vi "DSP 1st.vi"(0 "Input Signal":dbl[](array[numeric]), 1 "Work position parameter":i32[](array[numeric]), 2 "Minus Noise(F : Don't)":bool, 3 "Smooth(F : Don't)":bool, 5 "RF Window":dbl[](array[numeric]), 7 "IIR Filter Cluster":T1 caption="IIR滤波器簇" {"Forward Coefficients" format="%.4f"; "Reverse Coefficients" format="%.4f"}, 9 "Noise Signal":dbl[](array[numeric]), 11 "error in (no error)":errorcluster caption="错误输入（无错误）", 12 "SPAN":i32, 13 "Logarithmic Base":dbl) -> (4 "DSP signal":dbl[](array[numeric]), 15 "error out":errorcluster caption="错误输出")   [LabVIEW 2015, in "Digital Signal Processing.lvlib"]
uses:
  Digital Signal Processing.lvlib
  <vilib>/Analysis/2dsp.llb/1D Convolution (DBL).vi
  <vilib>/Analysis/baseanly.llb/IIR Cascade Filter (DBL).vi
  <vilib>/Analysis/NI_AALPro.lvlib
  <vilib>/Analysis/NI_AALBase.lvlib
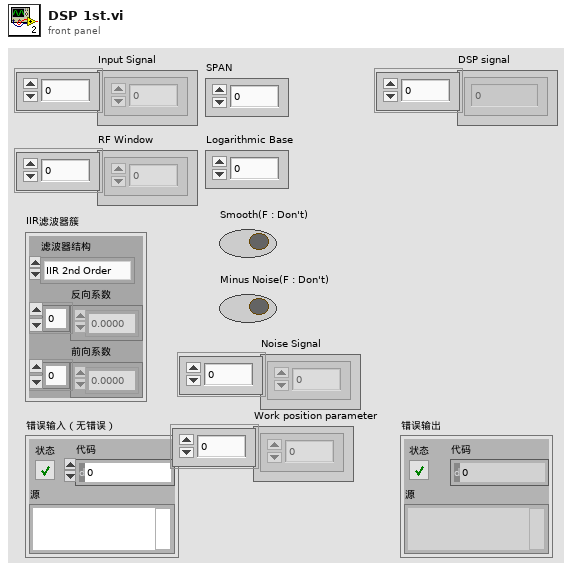
[diagram p1: front panel]
types:
  T1 = cluster{"filter structure":enum32{"IIR 2nd Order", "IIR 4th Order"}, "Reverse Coefficients":dbl[], "Forward Coefficients":dbl[]}
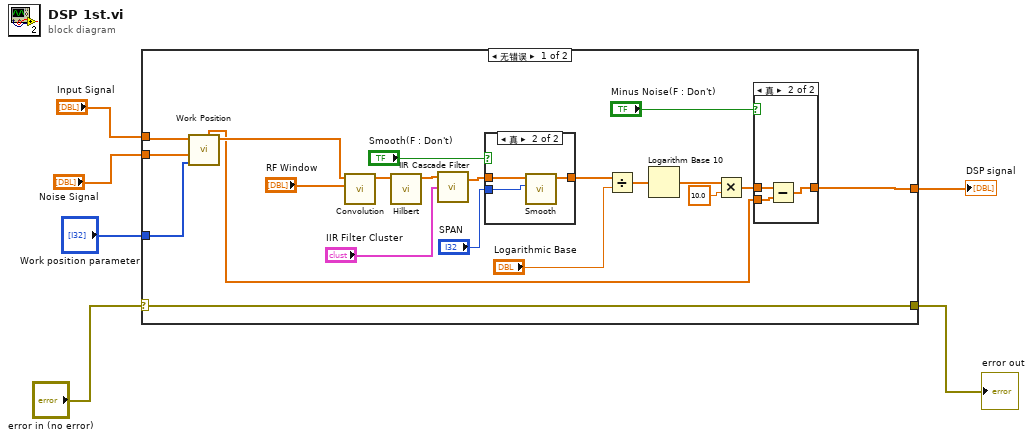
[diagram p0: block diagram]
diagram:
  n1 = case shown="无错误" "error in (no error)" {
    selector: "error in (no error)" -> [w12 w36]
    tunnel: "Input Signal" -> [w11 _]
    tunnel: [w13 _] -> w5
    tunnel: [w12 w36] -> w3
    tunnel: "Noise Signal" -> [w10 _]
    tunnel: "Work position parameter" -> [w7 _]
    frame No Error {
      n2 = call "Work Position.vi"("Work position parameter"=w7, "Noise"=w10, "S"=w11) -> ("S_1st_part"=w9:dbl[], "Noise_1st_part"=w8:dbl[])  [unwired: 3 in, 4 out]
      n3 = call-poly <vilib>:"Convolution.vi"("Y"="RF Window", "X"=w9) -> ("X * Y"=w17:dbl[])  [unwired: 1 in, 8 out]
      n4 = call "Hilbert.vi"("X"=w17) -> ("H(X)"=w16:dbl[])  [unwired: 10 in]
      n5 = call-poly <vilib>:"IIR Cascade Filter.vi"("IIR Filter Cluster"="IIR Filter Cluster", "X"=w16) -> ("Filtered X"=w15:dbl[])  [unwired: 1 in, 1 out]
      n6 = case shown="真" "Smooth(F : Don't)" {
        tunnel: w15 -> [w28 w31]
        tunnel: "SPAN" -> [_ w30]
        tunnel: [w28 w29] -> w18
        frame False {
        }
        frame True {
          n7 = call "Smooth.vi"("SPAN"=w30, "S"=w31) -> ("S_smooth"=w29:dbl[])  [unwired: 9 in]
        }
      }
      n8 = Divide(x=w18, y="Logarithmic Base") -> (x/y=w27:dbl[])
      n9 = Logarithm Base 10(1:w27) -> (0:w25:dbl[])
      n10 = Multiply(x=w25, y=10.0) -> (x*y=w19:dbl[])
      n11 = case shown="真" "Minus Noise(F : Don't)" {
        tunnel: w19 -> [w32 w35]
        tunnel: w8 -> [_ w34]
        tunnel: [w32 w33] -> w13
        frame False {
        }
        frame True {
          n12 = Subtract(x=w35, y=w34) -> (x-y=w33:dbl[])
        }
      }
    }
    frame Error {
    }
  }
  "DSP signal" <- w5
  "error out" <- w3
